vi "SV Limit Testing for Monitoring (1 Ch) (scalar) (DBL).vi"(7 "reset":bool, 9 "lower limit":dbl=-inf format="%.2f", 10 "upper limit":dbl=inf format="%.2f", 11 "input value":dbl=inf format="%.2f") -> (1 "lower limit clearance":dbl format="%.6f", 2 "upper limit clearance":dbl format="%.6f", 3 "test passed?":bool)   [LabVIEW 2017]
doc: "Performs limit testing on waveforms, spectra, XY data, identified peaks, or scalar measurements. You can wire <B>output values</B> to a graph to view the limits, signal, and failures. Wire data to the<B> signal in</B> input to determine the polymorphic instance to use or manually select the instance."
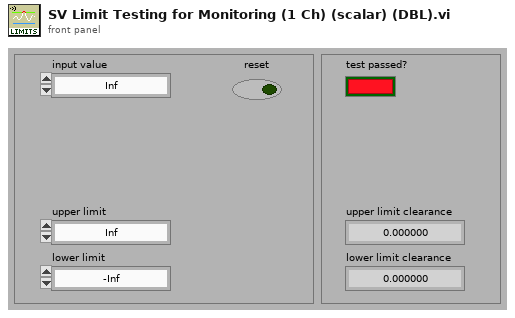
[diagram p1: front panel]
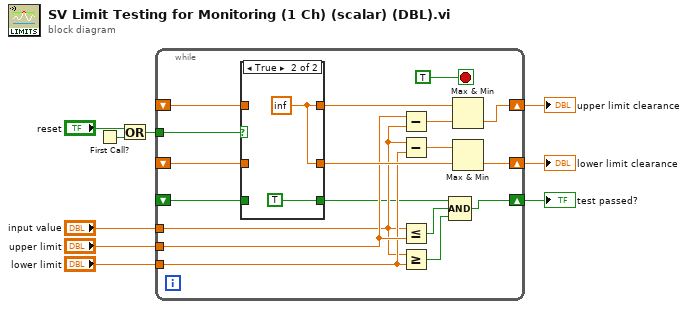
[diagram p0: block diagram]
diagram:
  n1 = First Call?() -> (First Call?: T/F=w1:bool)
  n2 = Or(x="reset", y=w1) -> (x .or. y?=w2:bool)
  n3 = while {
    tunnel: "input value" -> [w12]
    tunnel: "upper limit" -> [w19]
    tunnel: "lower limit" -> [w15]
    shift-right: [w27] -> w6
    shift-left: _ -> [w24]
    shift-right: [w26] -> w5
    shift-left: _ -> [w22]
    shift-right: [w11] -> w4
    shift-left: _ -> [w20]
    tunnel: w2 -> [w25]
    stop <- TRUE stop-if-true
    n4 = case shown="True" w25 {
      tunnel: w24 -> [w30 _]
      tunnel: [w30 w31] -> w23
      tunnel: w22 -> [w29 _]
      tunnel: [w29 w31] -> w21
      tunnel: w20 -> [w28 _]
      tunnel: [w28 TRUE] -> w10
      frame False {
      }
      frame True {
        w31 = inf
      }
    }
    n5 = Subtract(x=w19, y=w12) -> (x-y=w14:dbl)
    n6 = Subtract(x=w12, y=w15) -> (x-y=w13:dbl)
    n7 = Less Or Equal?(x=w12, y=w19) -> (x <= y?=w17:bool)
    n8 = Greater Or Equal?(x=w12, y=w15) -> (x >= y?=w16:bool)
    n9 = Compound Arithmetic op=AND(w10, w17, w16) -> (w11:bool)
    n10 = Max & Min(x=w23, y=w14) -> (min(x,y)=w27:dbl)  [unwired: 1 out]
    n11 = Max & Min(x=w13, y=w21) -> (min(x,y)=w26:dbl)  [unwired: 1 out]
  }
  "test passed?" <- w4
  "upper limit clearance" <- w6
  "lower limit clearance" <- w5
